vi "DraggingDresser.vi"() -> ()   [LabVIEW 2014]
panel:
  out "Force":dbl[](array[numeric])
  out "Angle for Minimum Force":i32 format="%.1f"
  in  "Coefficient of Kinetic Friction":dbl format="%.1f"
  out "Waveform Graph":dbl[](graph)
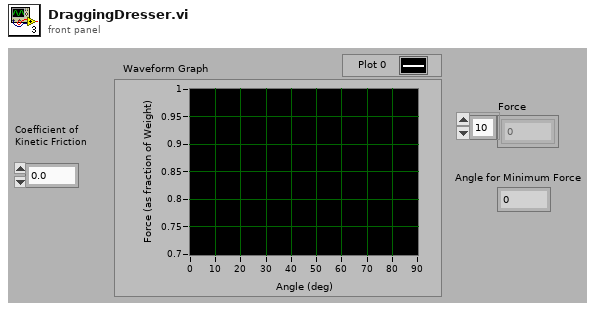
[diagram p1: front panel]
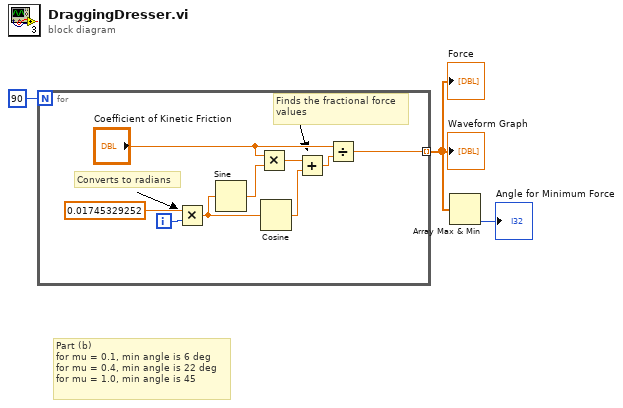
[diagram p0: block diagram]
diagram:
  # "Part (b)\nfor mu = 0.1, min angle is 6 deg\nfor mu = 0.4, min angle is 22 deg\nfor mu = 1.0, min angle is 45"
  n1 = for {
    N: 90 -> [_]
    tunnel: [w7] -> w2 mode=indexing
    i -> [w6]
    # "Converts to radians"
    # "Finds the fractional force\nvalues"
    n2 = Multiply(x=0.01745329252, y=w6) -> (x*y=w4:dbl)
    n3 = Sine(x=w4) -> (sin(x)=w11:dbl)
    n4 = Multiply(x="Coefficient of Kinetic Friction", y=w11) -> (x*y=w10:dbl)
    n5 = Cosine(x=w4) -> (cos(x)=w9:dbl)
    n6 = Add(x=w10, y=w9) -> (x+y=w8:dbl)
    n7 = Divide(x="Coefficient of Kinetic Friction", y=w8) -> (x/y=w7:dbl)
  }
  "Force" <- w2
  "Waveform Graph" <- w2
  n8 = Array Max & Min(array=w2) -> (min index (indices)=→"Angle for Minimum Force":i32)  [unwired: 3 out]
